vi "Write Pulse Recorder Configuration.vi"(8 "error in (no error)":errorcluster, 10 "Configuration":T1={"Post-trigger delay"=0.01, "Post-trigger duration"=0.1, "Rate"=1000000.0, "Ranges"=[10.0], "Re-name channels"=[], "Active channels"="0:1", "External clock"=FALSE} {"Rate" format="%#_8pHz"; "Post-trigger duration" format="%#_6ps"; "Post-trigger delay" format="%#_6ps"; "Ranges" format="%#_6pV"}, 11 "Lockin Digitizer in":refnum<class "Lockin Digitizer.lvclass">) -> (0 "error out":errorcluster, 3 "Lockin Digitizer out":refnum<class "Lockin Digitizer.lvclass">)   [LabVIEW 2021, in "Lockin Digitizer.lvclass"]
uses:
  Lockin Digitizer.lvclass
  NHMFL_Core/Libraries/Instruments/Pulse Driver/Pusle Driver Configuration.ctl
  Lockin Digitizer.lvclass/Lockin Digitizer.ctl
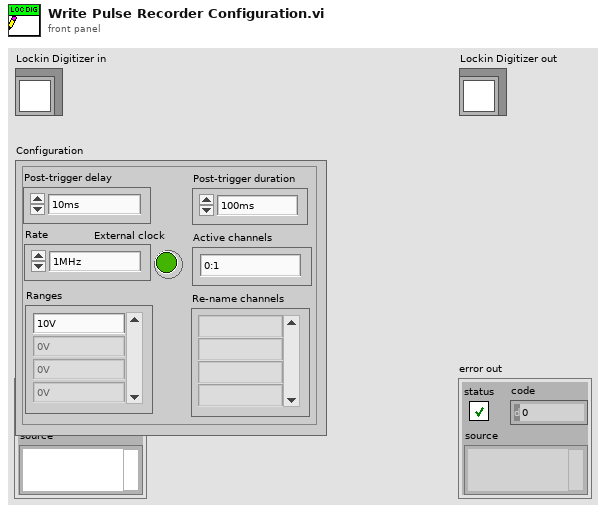
[diagram p1: front panel]
types:
  T1 = typedef "Pusle Driver Configuration.ctl" = cluster{"Post-trigger delay":dbl, "Post-trigger duration":dbl, "Rate":dbl, "Ranges":dbl[], "Re-name channels":string[], "Active channels":string, "External clock":bool}
  T2 = typedef "Lockin Digitizer Configuration.ctl" = cluster{"Post-trigger delay":dbl, "Post-trigger duration":dbl, "Rate":dbl, "Ranges":dbl[], "Re-name channels":string[], "Active channels":string, "External\nclock":bool, "Frequencies":dbl[], "Time\nconstant":dbl, "Output \namplitudes":dbl[], "Input\nchannles":string[]}
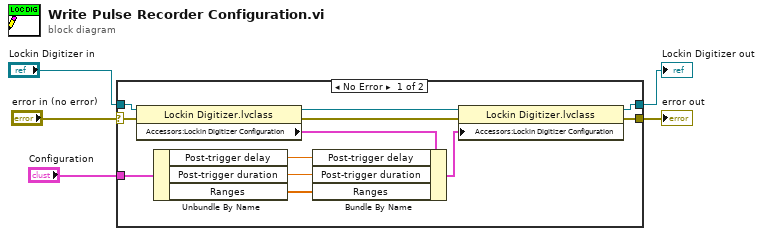
[diagram p0: block diagram]
diagram:
  n1 = case shown="No Error" "error in (no error)" {
    selector: "error in (no error)" -> [w11 w19]
    tunnel: [w13 w19] -> w4
    tunnel: "Lockin Digitizer in" -> [w15 w18]
    tunnel: "Configuration" -> [w10 _]
    tunnel: [w12 w18] -> w5
    frame No Error {
      n2 = property class="Lockin Digitizer.lvclass"(reference=w15, error in=w11) -> (reference out=w17:refnum<class "Lockin Digitizer.lvclass">, error out=w16:errorcluster, "Accessors:Lockin Digitizer Configuration"=w14:T2)
      n3 = Unbundle By Name(w10) -> ("Post-trigger delay"=w9:dbl, "Post-trigger duration"=w8:dbl, "Ranges"=w7:dbl[])
      n4 = Bundle By Name(cluster=w14, "Post-trigger delay"=w9, "Post-trigger duration"=w8, "Ranges"=w7) -> (w6:T2)
      n5 = property class="Lockin Digitizer.lvclass"(reference=w17, error in=w16, "Accessors:Lockin Digitizer Configuration"=w6) -> (reference out=w12:refnum<class "Lockin Digitizer.lvclass">, error out=w13:errorcluster)
    }
    frame Error {
    }
  }
  "error out" <- w4
  "Lockin Digitizer out" <- w5
